vi "Pixellate Lithography Data.vi"(8 "error in":errorcluster, 10 "Lithography Data":T3(array[cluster]), 11 "BigMAQ in":refnum<class "BigMAQ.lvclass">) -> (0 "error out":errorcluster, 2 "Array":T1[](array[typedef]), 3 "BigMAQ out":refnum<class "BigMAQ.lvclass">)   [LabVIEW 2019, in "BigMAQ.lvclass"]
uses:
  BigMAQ.lvclass
  <userlib>/LevyLab/Relay Box/Typedefs/Resistor--enum.ctl
  Overlay.ctl
  BigMAQ.lvclass/BigMAQ.ctl
  <userlib>/LevyLab/Relay Box/Relay-Box.lvclass
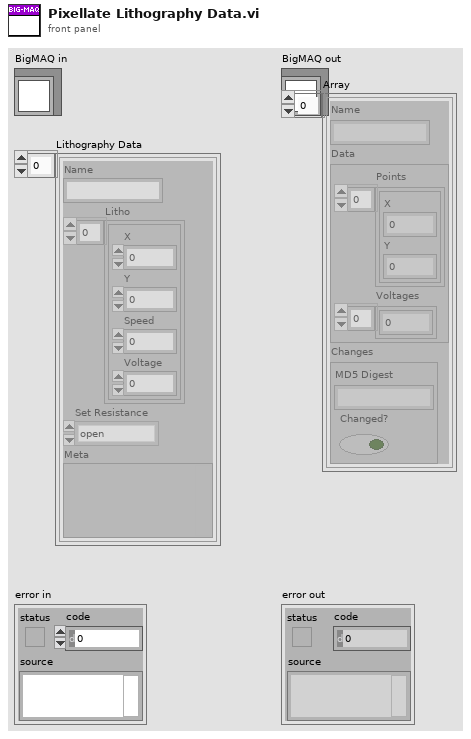
[diagram p1: front panel]
types:
  T1 = typedef "BigMAQ.lvclass/Overlay.ctl" = cluster{"Name":string, "Data":cluster{"Points":cluster{"X":dbl, "Y":dbl}[], "Voltages":dbl[]}, "Changes":cluster{"MD5 Digest":string, "Changed?":bool}}
  T2 = typedef "Relay-Box.lvclass/Resistor--enum.ctl" = enum16{"open", "discharge tip", "0 ohms", "100k ohm", "10M ohm", "1G ohm"}
  T3 = cluster{"Name":string, "Litho":cluster{"X":dbl, "Y":dbl, "Speed":dbl, "Voltage":dbl}[], "Set Resistance":T2, "Meta":variant}[]
  T4 = cluster{"X":dbl, "Y":dbl, "Speed":dbl, "Voltage":dbl}
  T5 = cluster{"X":dbl, "Y":dbl, "Speed":dbl, "Voltage":dbl}[]
  T6 = cluster{"X":bool, "Y":bool, "Speed":bool, "Voltage":bool}
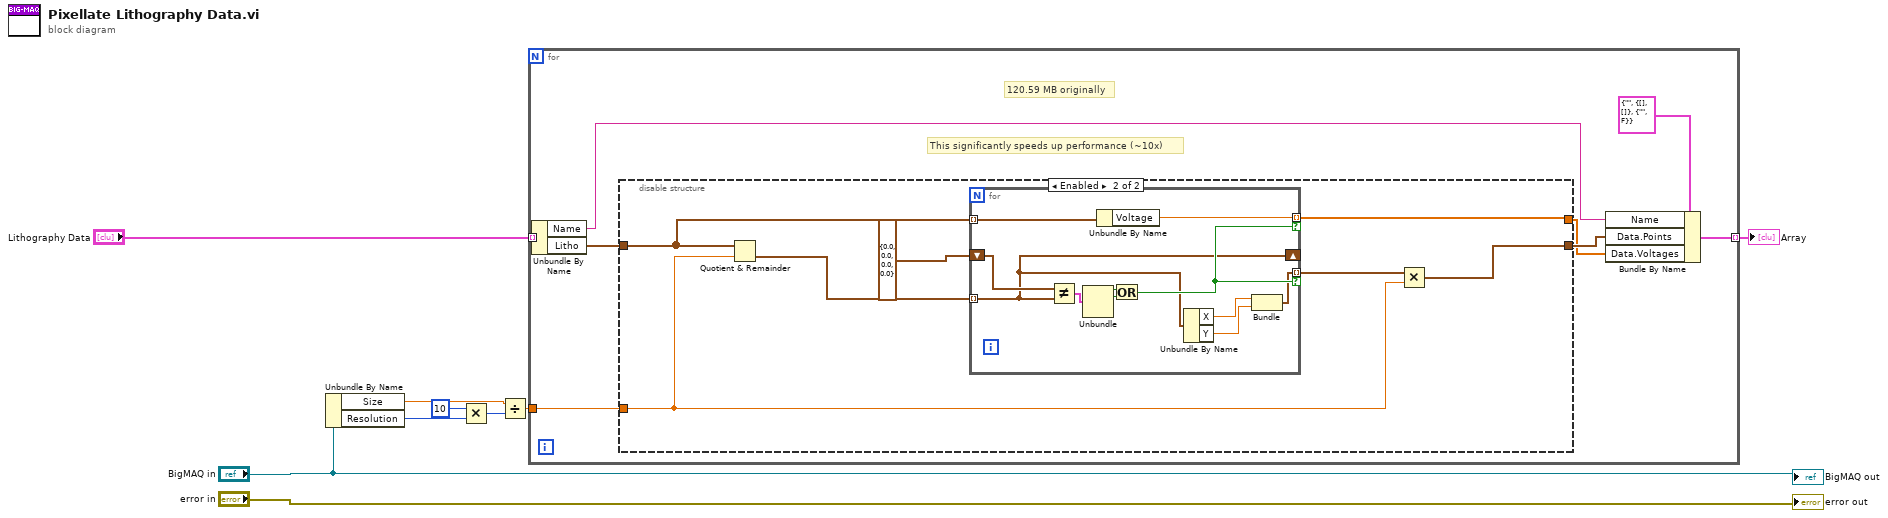
[diagram p0: block diagram]
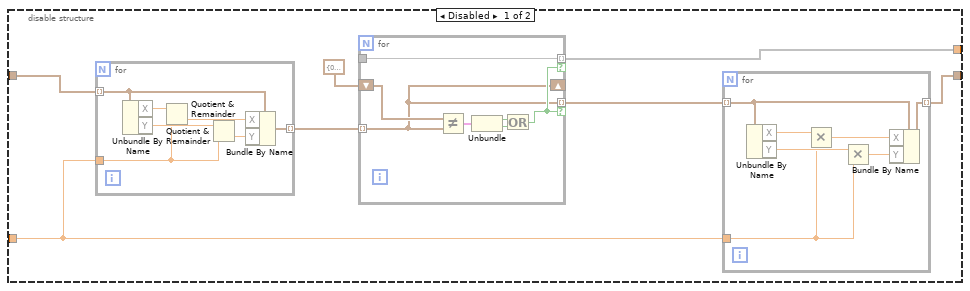
[diagram p2: hidden frame]
diagram:
  n1 = Unbundle By Name("BigMAQ in") -> ("Size"=w5:dbl, "Resolution"=w6:i32)
  n2 = Multiply(x=10, y=w6) -> (x*y=w8:i32)
  n3 = Divide(x=w5, y=w8) -> (x/y=w7:dbl)
  n4 = for {
    tunnel: w7 -> [w16]
    tunnel: "Lithography Data" -> [w11] mode=indexing
    tunnel: [w10] -> w1 mode=indexing
    # "120.59 MB originally"
    # "This significantly speeds up performance (~10x)"
    n5 = Unbundle By Name(w11) -> ("Name"=w12:string, "Litho"=w17:T5)
    n6 = disable-structure shown="Enabled" {
      disable-tunnel: w17 -> [w25 w49]
      disable-tunnel: [w22 w50] -> w14
      disable-tunnel: [w20 w47] -> w13
      disable-tunnel: w16 -> [w18 w51]
      frame Disabled {
        n7 = for {
          tunnel: w25 -> [w36] mode=indexing
          tunnel: [w37] -> w23 mode=indexing
          tunnel: w18 -> [w33]
          n8 = Unbundle By Name(w36) -> ("X"=w34:dbl, "Y"=w35:dbl)
          n9 = Quotient & Remainder(x=w34, y=w33) -> (floor(x/y)=w39:dbl)  [unwired: 1 out]
          n10 = Quotient & Remainder(x=w35, y=w33) -> (floor(x/y)=w38:dbl)  [unwired: 1 out]
          n11 = Bundle By Name(cluster=w36, "X"=w39, "Y"=w38) -> (w37:T4)
        }
        n12 = for {
          shift-right: [w40] -> _
          shift-left: cluster{"X":dbl, "Y":dbl} {"X"=0.0, "Y"=0.0} ("Litho Point") -> [w46]
          tunnel: [w40] -> w21 mode=indexing if=w41
          tunnel: w23 -> [w40] mode=indexing
          tunnel: [w42] -> w19
          tunnel: [w42] -> w20 mode=indexing if=w41
          n13 = Not Equal?(x=w46, y=w40) -> (x != y?=w45:cluster{"X":bool, "Y":bool})
          n14 = Unbundle(w45) -> ("X"=w44:bool, "Y"=w43:bool)
          n15 = Or(x=w44, y=w43) -> (x .or. y?=w41:bool)
        }
        n16 = for {
          tunnel: [w26] -> w22 mode=indexing
          tunnel: w21 -> [w31] mode=indexing
          tunnel: w18 -> [w27]
          n17 = Unbundle By Name(w31) -> ("X"=w32:dbl, "Y"=w28:dbl)
          n18 = Multiply(x=w32, y=w27) -> (x*y=w30:dbl)
          n19 = Multiply(x=w28, y=w27) -> (x*y=w29:dbl)
          n20 = Bundle By Name(cluster=w31, "X"=w30, "Y"=w29) -> (w26:T4)
        }
      }
      frame Enabled {
        n21 = Quotient & Remainder(x=w49, y=w51) -> (floor(x/y)=w53:T5)  [unwired: 1 out]
        n22 = for {
          shift-right: [w54] -> _
          shift-left: T4 {"X"=0.0, "Y"=0.0, "Speed"=0.0, "Voltage"=0.0} ("Litho Point") -> [w64]
          tunnel: [w55] -> w52 mode=indexing if=w58
          tunnel: w53 -> [w54] mode=indexing
          tunnel: w49 -> [w60] mode=indexing
          tunnel: [w59] -> w47 mode=indexing if=w58
          n23 = Not Equal?(x=w64, y=w54) -> (x != y?=w63:T6)
          n24 = Unbundle(w63) -> ("X"=w62:bool, "Y"=w61:bool)  [unwired: 2 out]
          n25 = Unbundle By Name(w60) -> ("Voltage"=w59:dbl)
          n26 = Or(x=w62, y=w61) -> (x .or. y?=w58:bool)
          n27 = Unbundle By Name(w54) -> ("X"=w57:dbl, "Y"=w56:dbl)
          n28 = Bundle("X"=w57, "Y"=w56) -> (w55:cluster{"X":dbl, "Y":dbl})  [unwired: 1 in]
        }
        n29 = Multiply(x=w52, y=w51) -> (x*y=w50:cluster{"X":dbl, "Y":dbl}[])
      }
    }
    n30 = Bundle By Name(cluster=T1 {"Name"="", "Data"={"Points"=[], "Voltages"=[]}, "Changes"={"MD5 Digest"="", "Changed?"=FALSE}} ("Pixellated Overlay"), "Name"=w12, "Data.Points"=w14, "Data.Voltages"=w13) -> (w10:T1)
  }
  "Array" <- w1
  "error out" <- "error in"
  "BigMAQ out" <- "BigMAQ in"
